vi "Show_scanners.vi"(8 "error in":errorcluster, 10 "Min/Max Voltage":dbl=1.0 format="%0.2f", 11 "task/channels in":refnum<k21>) -> (0 "error out":errorcluster, 3 "task out":refnum<k21>)   [LabVIEW 2018]
uses:
  <vilib>/Analysis/1siggen.llb/Ramp Pattern by Samples.vi
  <vilib>/DAQmx/write.llb/DAQmx Write (Analog 2D DBL NChan NSamp).vi
  <vilib>/DAQmx/configure/timing.llb/DAQmx Timing (Sample Clock).vi
  <vilib>/DAQmx/miscellaneous.llb/DAQmx Fill In Error Info.vi
  <vilib>/Analysis/NI_AALBase.lvlib
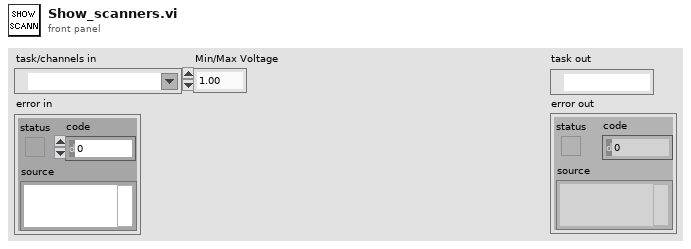
[diagram p1: front panel]
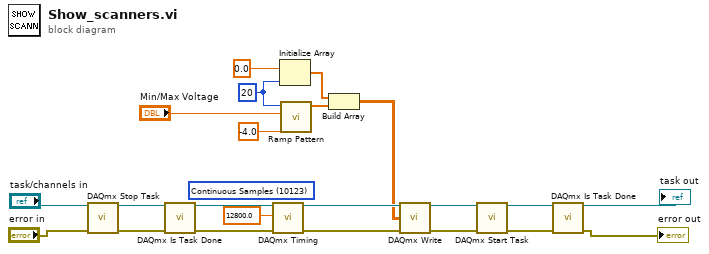
[diagram p0: block diagram]
diagram:
  w17 = 20 ("dimension size")
  (unwired) 10123 items=["Finite Samples"=10178, "Continuous Samples"=10123, "Hardware Timed Single Point"=12522] ("sample mode")
  n1 = call <vilib>:"DAQmx Stop Task.vi"("task/channels in"="task/channels in", "error in"="error in") -> ("task out"=w7:refnum<k21>, "error out"=w6:errorcluster)  [unwired: 12 in]
  n2 = call <vilib>:"DAQmx Is Task Done.vi"("task/channels in"=w7, "error in"=w6) -> ("task out"=w4:refnum<k21>, "error out"=w2:errorcluster)  [unwired: 11 in, 1 out]
  n3 = call-poly <vilib>:"DAQmx Timing.vi"("task/channels in"=w4, "rate"=12800.0, "error in"=w2) -> ("task out"=w22:refnum<k21>, "error out"=w20:errorcluster)  [unwired: 11 in]
  n4 = Initialize Array(0.0 ("element"), w17) -> (w19:dbl[])
  n5 = call-poly <vilib>:"Ramp Pattern.vi"("start"=-4.0, "end"="Min/Max Voltage", "samples"=w17) -> ("Ramp Pattern"=w18:dbl[])  [unwired: 7 in, 1 out]
  n6 = Build Array(w19, w18) -> (w15:dbl[][])
  n7 = call-poly <vilib>:"DAQmx Write.vi"("task/channels in"=w22, "data"=w15, "error in"=w20) -> ("task out"=w14:refnum<k21>, "error out"=w13:errorcluster)  [unwired: 10 in, 1 out]
  n8 = call <vilib>:"DAQmx Start Task.vi"("task/channels in"=w14, "error in"=w13) -> ("task out"=w9:refnum<k21>, "error out"=w8:errorcluster)  [unwired: 12 in]
  n9 = call <vilib>:"DAQmx Is Task Done.vi"("task/channels in"=w9, "error in"=w8) -> ("task out"=→"task out":refnum<k21>, "error out"=→"error out":errorcluster)  [unwired: 11 in, 1 out]
